vi "Init_Control.vi"(8 "error in (no error)":errorcluster) -> (0 "error out":errorcluster, 1 "App.SaveVersions":string[](array[string]), 2 "Styles strings":string[](array[string]), 3 "Control out":refnum<class "Control.lvclass">)   [LabVIEW 2012, in "Control.lvclass"]
doc: "Instantiates a new object based on the Control class."
uses:
  Control.lvclass
  Typedefs/TypeDef_Action.ctl
  <userlib>/BitMan/BitMap class/BitMap.lvclass
  Controls/_ui_tools_font.ctl
  Controls/BX.Orientation__LCR _Modified.ctl
  Control.lvclass/Control.ctl
  <userlib>/_OpenG.lib/file/file.llb/Build Path - Traditional - path__ogtk.vi
  <userlib>/_OpenG.lib/array/array.llb/Conditional Auto-Indexing Tunnel (String)__ogtk.vi
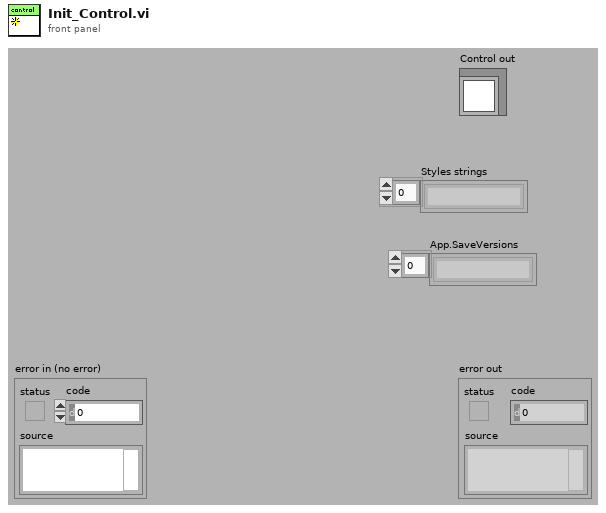
[diagram p1: front panel]
types:
  T1 = typedef "Control.lvclass/BX.Orientation__LCR _Modified.ctl" = u8
  T2 = typedef "Control.lvclass/_ui_tools_font.ctl" = cluster{"Font Name:":string, "Size":i16, "Strikeout?":bool, "Italic?":bool, "Underline?":bool, "Outline?":bool, "Shadow?":bool, "Bold?":bool}
  T3 = typedef "Control.lvclass/TypeDef_Action.ctl" = u16
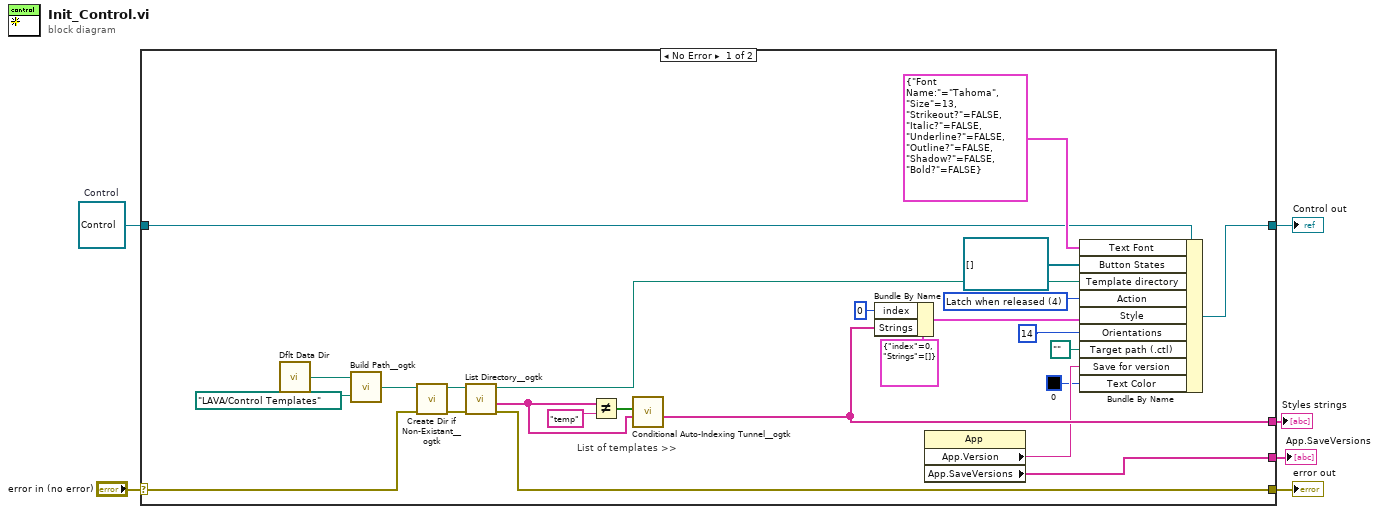
[diagram p0: block diagram]
diagram:
  w2 = refnum<class "Control.lvclass"> refnum  # Control
  n1 = case shown="No Error" "error in (no error)" {
    selector: "error in (no error)" -> [w12 w33]
    tunnel: [w11 w33] -> w6
    tunnel: [w31 w32] -> w5
    tunnel: w2 -> [w20 w32]
    tunnel: [w19 _] -> w4
    tunnel: [w9 _] -> w1
    frame No Error {
      w10 = T3 4 items=["Switch when pressed", "Switch when released", "Switch until release", "Latch when pressed", "Latch when released", "Latch until released"] ("Action")
      # "List of templates >>"
      n2 = call <vilib>:"Dflt Data Dir.vi"() -> ("App:Default Data Directory"=w16:path)
      n3 = call-poly <userlib>:"Build Path__ogtk.vi"("name or relative path"=path "LAVA/Control Templates" ("Relative path (.)"), "base path"=w16) -> ("appended path"=w15:path)
      n4 = call <userlib>:"Create Dir if Non-Existant__ogtk.vi"("error in (no error)"=w12, "Directory Path"=w15) -> ("error out"=w13:errorcluster, "dup Directory Path"=w14:path)  [unwired: 1 in, 7 out]
      n5 = call <userlib>:"List Directory__ogtk.vi"("error in (no error)"=w13, "directory path"=w14) -> ("error out"=w11:errorcluster, "directory names"=w25:string[], "dup directory path"=w24:path)  [unwired: 1 in, 2 out]
      n6 = Not Equal?(x=w25, y="temp") -> (x != y?=w26:bool[])
      n7 = call-poly <userlib>:"Conditional Auto-Indexing Tunnel__ogtk.vi"("Array in"=w25, "Elements to keep"=w26) -> ("Filtered Array out"=w19:string[])  [unwired: 5 out]
      n8 = Bundle By Name(cluster=cluster{"index":u16, "Strings":string[]} {"index"=0, "Strings"=[]} ("Style"), "index"=u16 0, "Strings"=w19) -> (w30:cluster{"index":u16, "Strings":string[]})
      n9 = property class="App"() -> ("App.Version"=w8:string, "App.SaveVersions"=w9:string[])  [unwired: 2 in, 2 out]
      n10 = Bundle By Name(cluster=w20, "Text Font"=T2 {"Font Name:"="Tahoma", "Size"=13, "Strikeout?"=FALSE, "Italic?"=FALSE, "Underline?"=FALSE, "Outline?"=FALSE, "Shadow?"=FALSE, "Bold?"=FALSE} ("Font"), "Button States"=refnum<class "BitMap.lvclass">[] [], "Template directory"=w24, "Action"=w10, "Style"=w30, "Orientations"=T1 14, "Target path (.ctl)"=path "", "Save for version"=w8, "Text Color"=u32 0) -> (w31:refnum<class "Control.lvclass">)
    }
    frame Error {
    }
  }
  "error out" <- w6
  "Control out" <- w5
  "Styles strings" <- w4
  "App.SaveVersions" <- w1
